vi "SUB-ROM Data convert to table.vi"(4 "ROM Table Ref":refnum<vi>, 5 "ROM Data Ref":refnum<vi>) -> (1 "ROM Table":string[][](table)=[["Device ID", "1 (00000001h)", "MAX Value: 4294967295 (FFFFFFFFh)"], ["YEAR", "2 (02h)", "Year: 2002, MAX Value: 255 (FFh)"], ["Month", "3 (03h)", "Month:  3, MAX Value: 255 (FFh)"], ["Day", "4 (04h)", "Day:  4, MAX Value: 255 (FFh)"], ["Device Type", "5 (0005h)", "-"], ["Manufacturer ID", "6 (00000006h)", "MAX Value: 4294967295 (FFFFFFFFh)"], ["Cal_Scale A", "7 (07h)", "MAX Value: 255 (FF)"], ["Cal_Scale B", "8 (08h)", "MAX Value: 255 (FF)"], ["Cal_Acc. X", "9 (0009h)", "-"], ["Cal_Acc. Y", "10 (000Ah)", "-"], ["Cal_Acc. Z", "11 (000Bh)", "-"], ["Cal_Gy. X", "12 (000Ch)", "-"], ["Cal_Gy. Y", "13 (000Dh)", "-"], ["Cal_Gy. Z", "14 (000Eh)", "-"], ["Cal_Vol H", "15 (000Fh)", "-"], ["Cal_Vol L", "16 (0010h)", "-"], ["Cal_CDC Off 1", "17 (11h)", "-"], ["Cal_CDC Off 2", "18 (12h)", "-"], ["Cal_CDC Off 3", "19 (13h)", "-"], ["Cal_CDC Off 4", "20 (14h)", "-"], ["Cal_CDC Off 5", "21 (15h)", "-"], ["Cal_CDC Off 6", "22 (16h)", "-"], ["Cal_CDC Off 7", "23 (17h)", "-"], ["Cal_CDC Off 8", "24 (18h)", "-"], ["Firmware Revision", "25 (19h)", "-"], ["Operative Side", "26 (1Ah)", "-"], ["Cal_Compart. A_10", "27 (0000001Bh)", "-"], ["Cal_Compart. B_10", "28 (0000001Ch)", "-"], ["Reserved", "29 (1Dh)", "-"], ["Cal_Compart. A_11", "30 (0000001Eh)", "-"], ["Cal_Compart. B_11", "31 (0000001Fh)", "-"], ["Cal_Compart. A_12", "32 (00000020h)", "-"], ["Cal_Compart. B_12", "33 (00000021h)", "-"], ["Cal_Compart. A_13", "34 (00000022h)", "-"], ["Cal_Compart. B_13", "35 (00000023h)", "-"], ["Cal_Compart. A_14", "36 (00000024h)", "-"], ["Cal_Compart. B_14", "37 (00000025h)", "-"], ["Cal_Compart. A_16", "38 (00000026h)", "-"], ["Cal_Compart. B_16", "39 (00000027h)", "-"], ["Reserved", "40 (28h)", "-"], ["Acc. X_0 value", "41 (0029h)", "-"], ["Acc. Y_0 value", "42 (002Ah)", "-"], ["Acc. Z_0 value", "43 (002Bh)", "-"], ["Acc. X_45 value", "44 (002Ch)", "-"], ["Acc. Y_45 value", "45 (002Dh)", "-"], ["Acc. Z_45 value", "46 (002Eh)", "-"], ["Reserved", "47 (2Fh)", "-"], ["Acc. X_90 value", "48 (0030h)", "-"], ["Acc. Y_90 value", "49 (0031h)", "-"], ["Acc. Z_90 value", "50 (0032h)", "-"], ["Acc. X_180 value", "51 (0033h)", "-"], ["Acc. Y_180 value", "52 (0034h)", "-"], ["Acc. Z_180 value", "53 (0035h)", "-"], ["Second counter", "16 (0000h)", "-"], ["Reserved", "54 (36h)", "-"], ["", "", ""], ["", "", ""], ["", "", ""], ["", "", ""], ["", "", ""], ["", "", ""], ["", "", ""], ["", "", ""], ["", "", ""], ["", "", ""], ["", "", ""], ["", "", ""], ["", "", ""], ["", "", ""], ["", "", ""]], 2 "ROM Data":T1(array[cluster])=[{"RxOK"=TRUE, "ROM Data"=[0, 0, 0, 1, 2, 3, 4, 0, 5, 0, 0, 0, 6, 7, 8, 131, 2], "Index"=0}, {"RxOK"=TRUE, "ROM Data"=[0, 9, 0, 10, 0, 11, 0, 12, 0, 13, 0, 14, 0, 15, 0, 136, 5], "Index"=1}, {"RxOK"=TRUE, "ROM Data"=[0, 17, 0, 18, 0, 19, 0, 20, 0, 21, 0, 22, 0, 23, 0, 145, 8], "Index"=2}, {"RxOK"=TRUE, "ROM Data"=[25, 26, 0, 0, 0, 27, 0, 0, 0, 28, 29, 0, 0, 0, 0, 146, 11], "Index"=3}, {"RxOK"=TRUE, "ROM Data"=[25, 26, 0, 0, 0, 27, 0, 0, 0, 28, 29, 0, 0, 0, 0, 146, 14], "Index"=4}, {"RxOK"=TRUE, "ROM Data"=[25, 26, 0, 0, 0, 27, 0, 0, 0, 28, 29, 0, 0, 0, 0, 146, 17], "Index"=5}, {"RxOK"=TRUE, "ROM Data"=[25, 26, 0, 0, 0, 27, 0, 0, 0, 28, 29, 0, 0, 0, 0, 146, 20], "Index"=6}, {"RxOK"=TRUE, "ROM Data"=[25, 26, 0, 0, 0, 27, 0, 0, 0, 28, 29, 0, 0, 0, 0, 146, 23], "Index"=7}, {"RxOK"=TRUE, "ROM Data"=[25, 26, 0, 0, 0, 27, 0, 0, 0, 28, 29, 0, 0, 0, 0, 146, 26], "Index"=8}] {"Index" format="%02x"; "ROM Data" format="%02x"})   [LabVIEW 2015]
panel:
  out "Last Index":i32=8
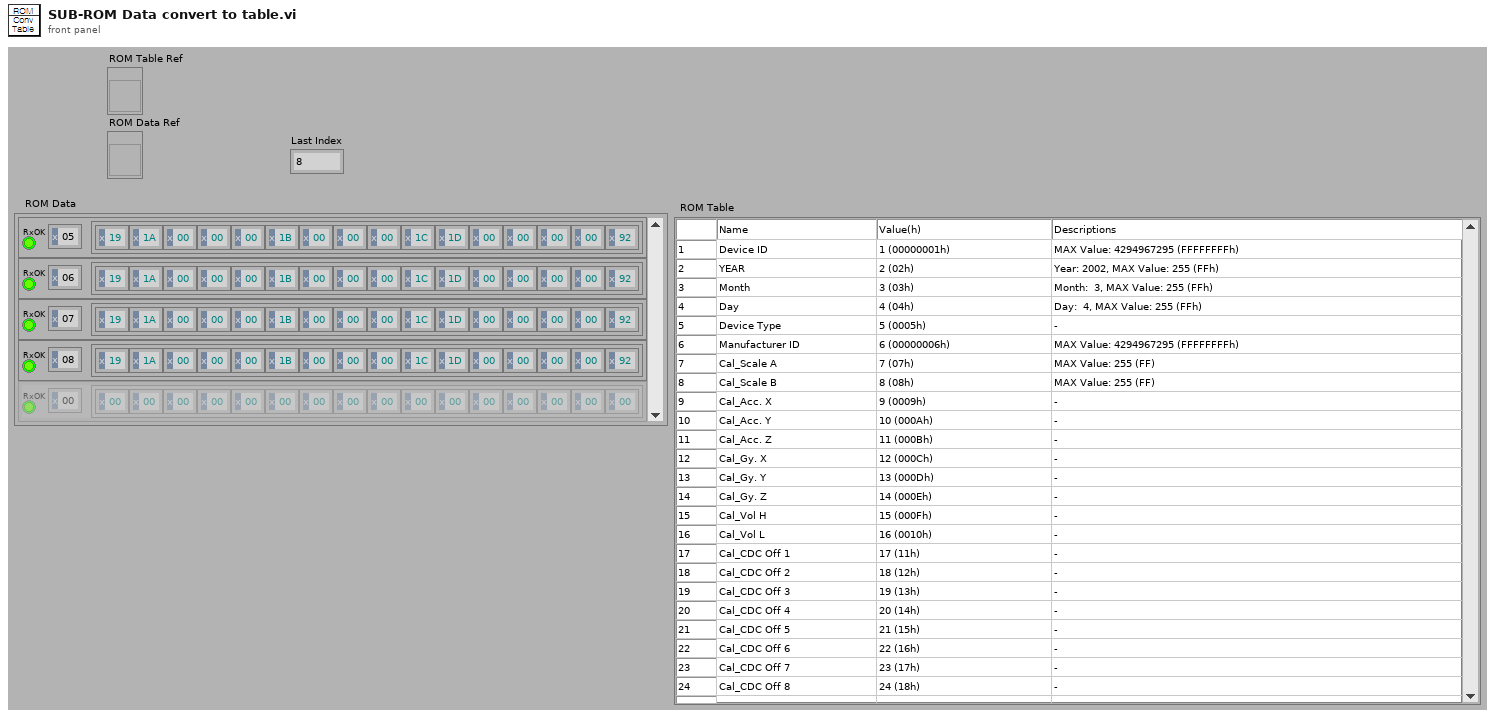
[diagram p1: front panel]
types:
  T1 = cluster{"RxOK":bool, "ROM Data":u8[], "Index":u8}[]
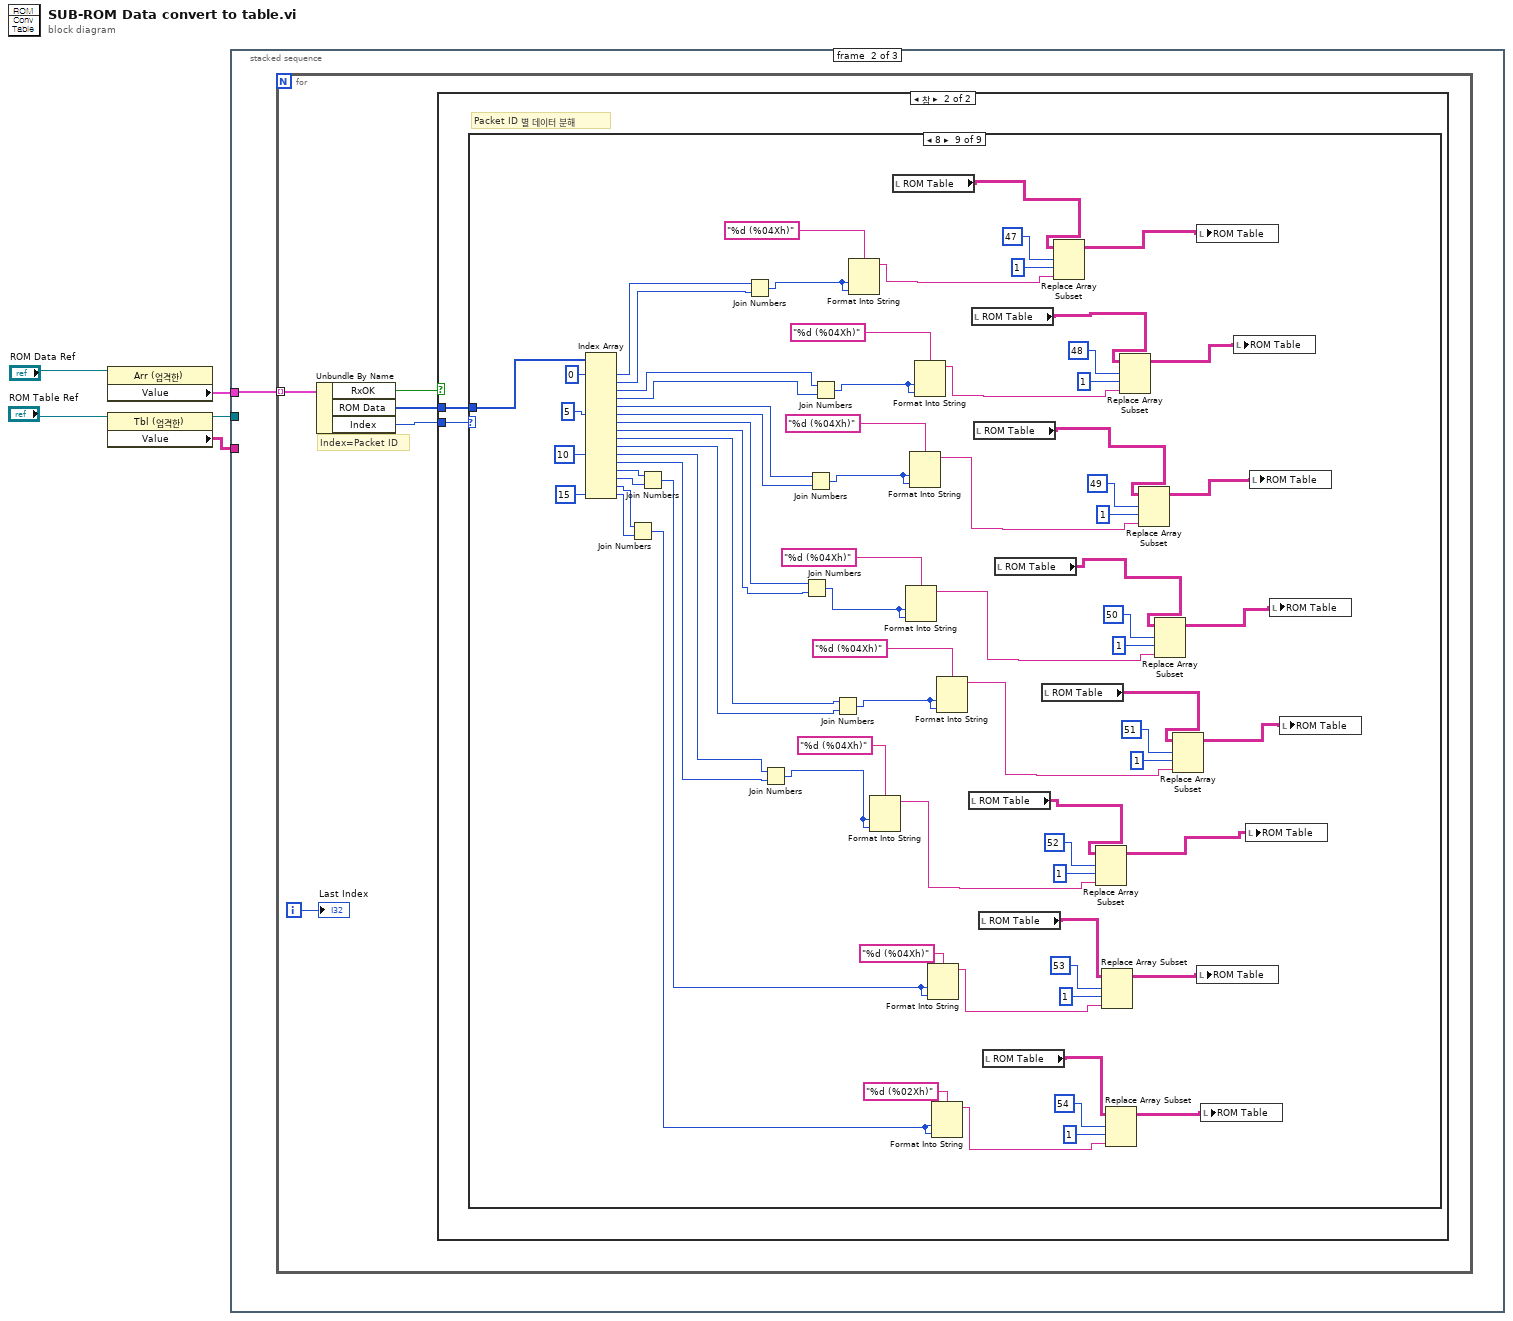
[diagram p0: block diagram]
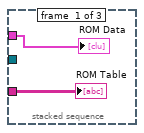
[diagram p2: hidden frame]
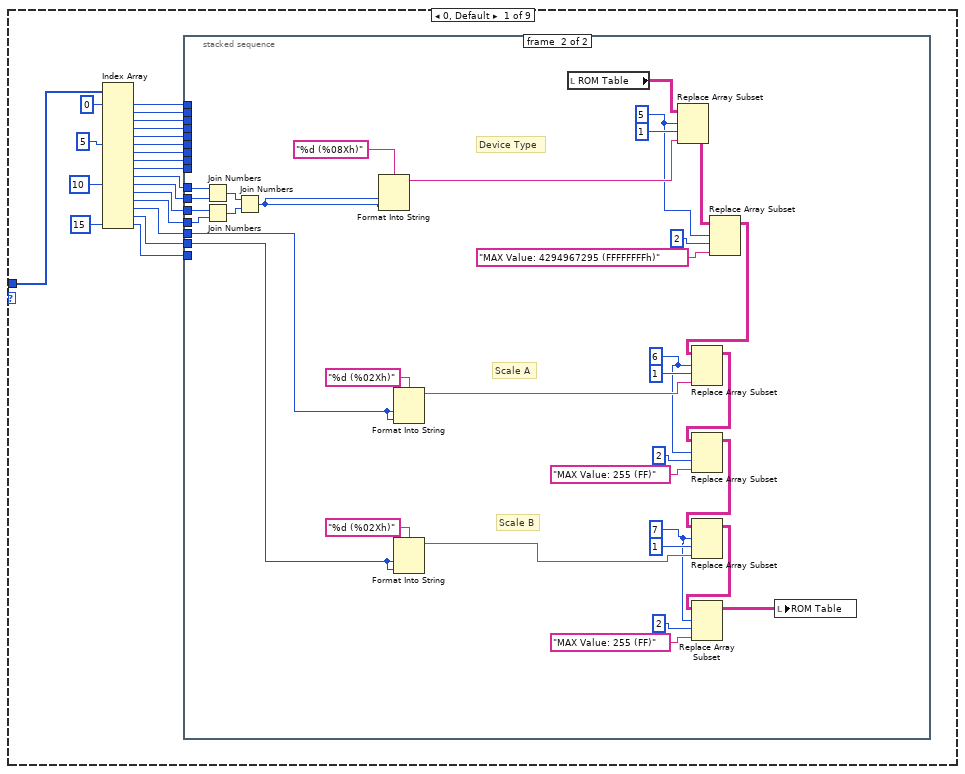
[diagram p4: hidden frame]
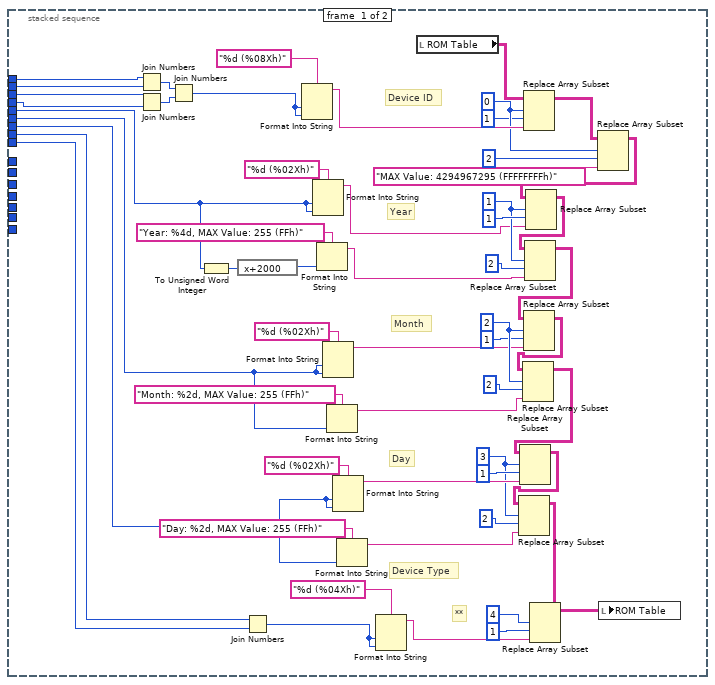
[diagram p5: hidden frame]
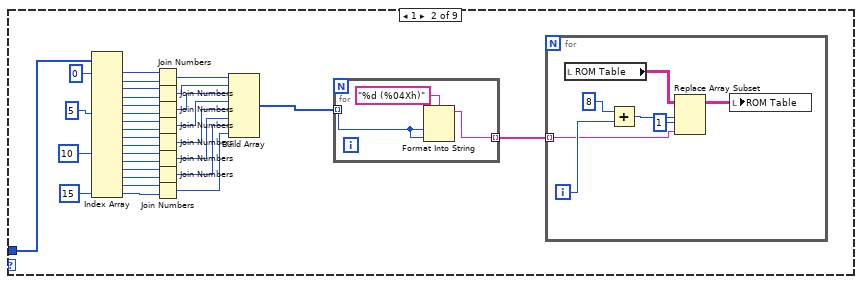
[diagram p6: hidden frame]
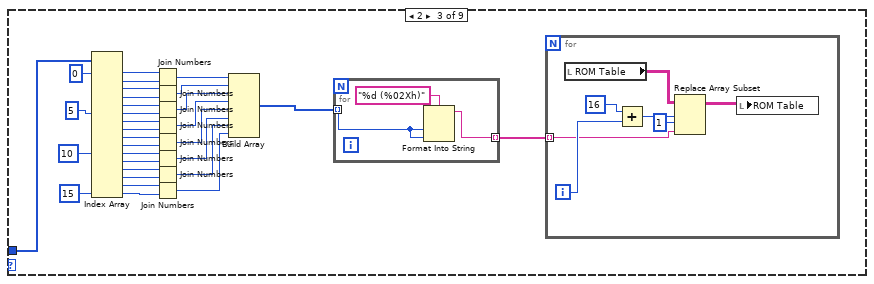
[diagram p7: hidden frame]
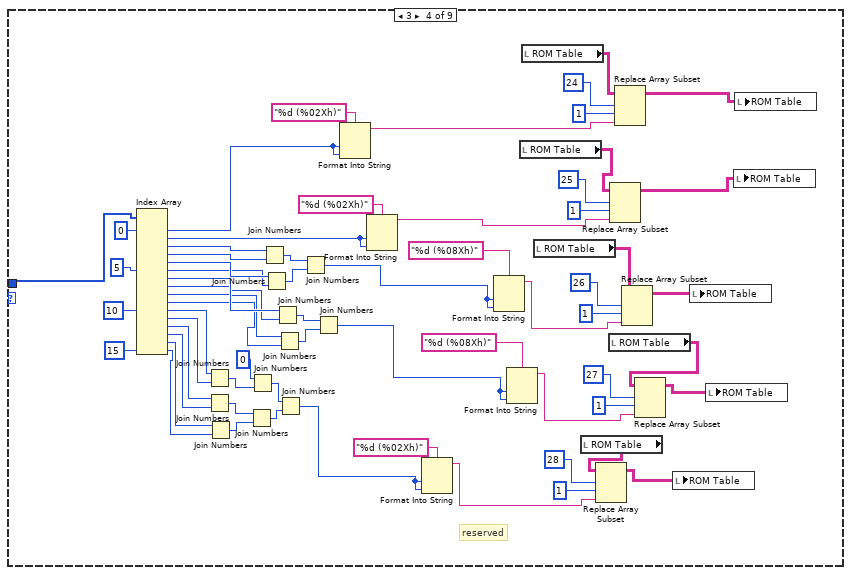
[diagram p8: hidden frame]
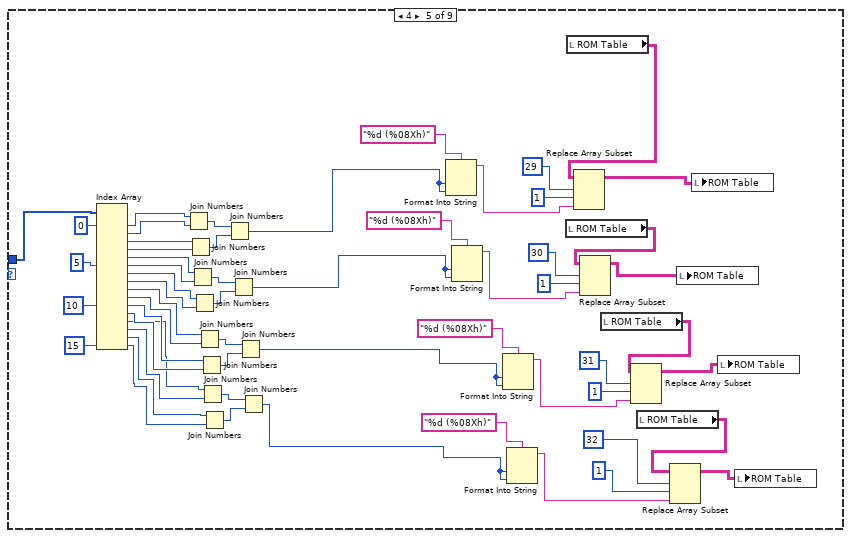
[diagram p9: hidden frame]
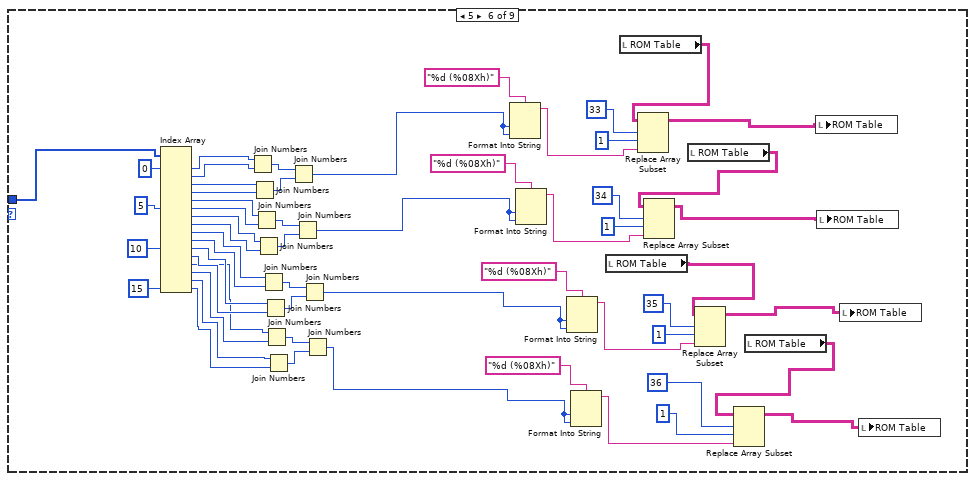
[diagram p10: hidden frame]
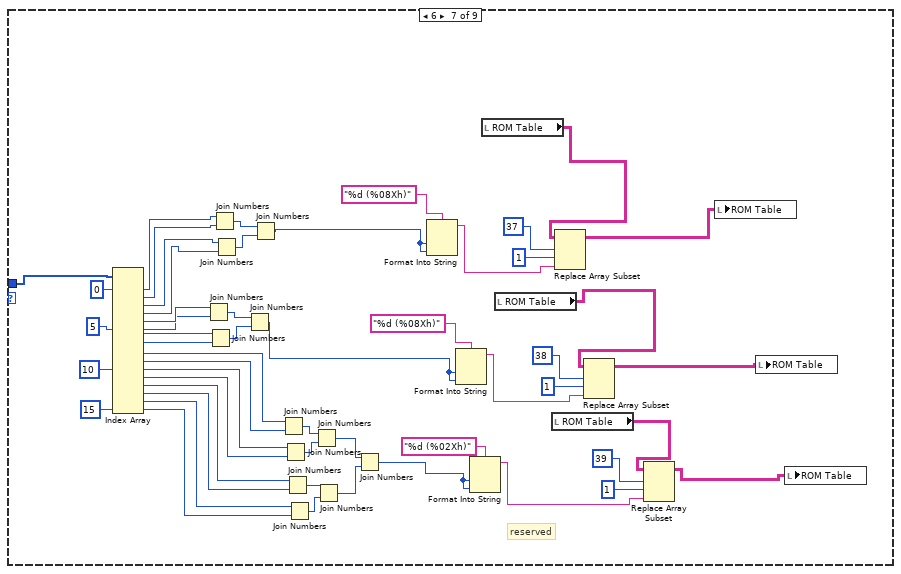
[diagram p11: hidden frame]
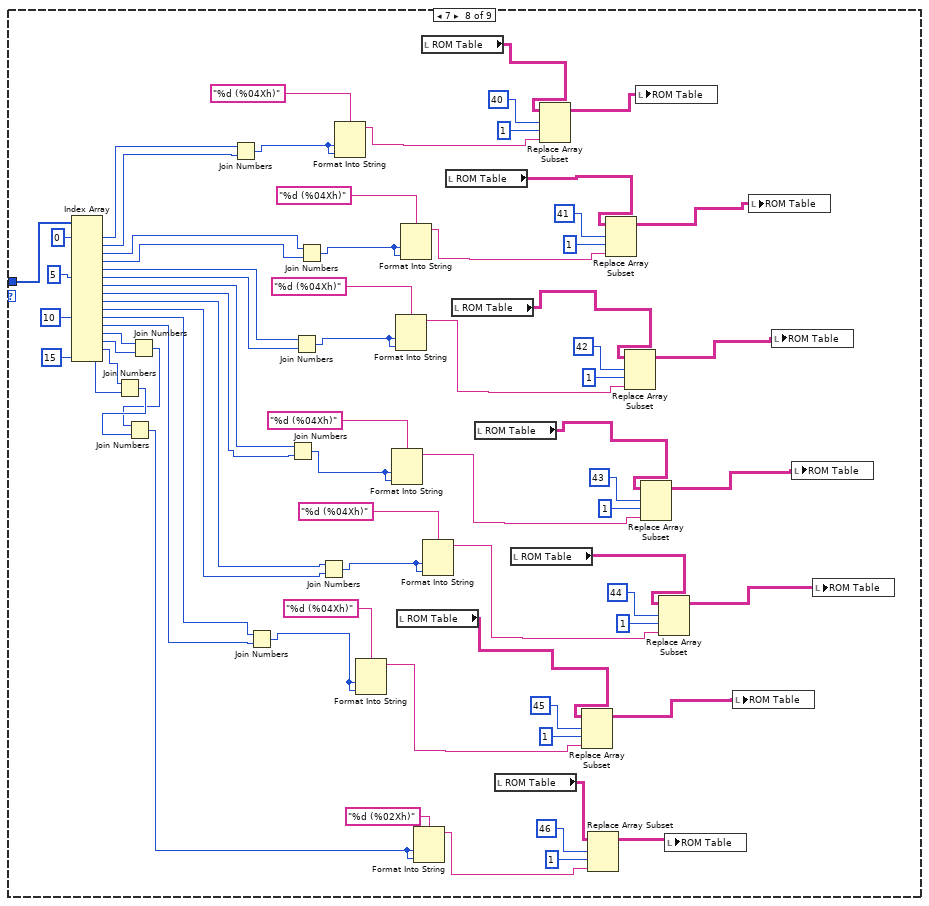
[diagram p12: hidden frame]
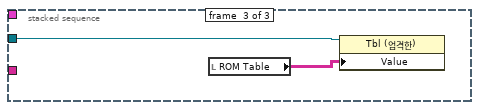
[diagram p13: hidden frame]
diagram:
  n1 = property class="Arr (엄격한)"(reference="ROM Data Ref") -> ("Value"=w3:T1)  [unwired: 1 in, 2 out]
  n2 = property class="Tbl (엄격한)"(reference="ROM Table Ref") -> (reference out=w1:refnum<vi>, "Value"=w2:string[][])  [unwired: 1 in, 1 out]
  n3 = stacked-sequence {
    tunnel: w3 -> [w7 w8 _]
    tunnel: w2 -> [w6 _ _]
    tunnel: w1 -> [_ _ w589]
    frame #0 {
      "ROM Data" <- w7
      "ROM Table" <- w6
    }
    frame #1 {
      n4 = for {
        tunnel: w8 -> [w13] mode=indexing
        i -> [w9]
        # "Index=Packet ID"
        n5 = Unbundle By Name(w13) -> ("RxOK"=w11:bool, "ROM Data"=w10:u8[], "Index"=w12:u8)
        n6 = case shown="참" w11 {
          tunnel: w12 -> [_ w15]
          tunnel: w10 -> [_ w14]
          frame False {
          }
          frame True {
            # "Packet ID 별 데이터 분해"
            n7 = case shown="8" w15 {
              tunnel: w14 -> [w32 w153 w194 w268 w325 w338 w434 w506 w537]
              frame 0, Default {
                n8 = Index Array(array=w32, index #1=0 ("인덱스"), index #6=5 ("인덱스"), index #11=10 ("인덱스"), index #16=15 ("인덱스")) -> (element #1=w31:u8, element #2=w30:u8, element #3=w29:u8, element #4=w28:u8, element #5=w27:u8, element #6=w26:u8, element #7=w25:u8, element #8=w24:u8, element #9=w23:u8, element #10=w22:u8, element #11=w21:u8, element #12=w20:u8, element #13=w19:u8, element #14=w18:u8, element #15=w17:u8, element #16=w16:u8)  [unwired: 12 in]
                n9 = stacked-sequence {
                  tunnel: w31 -> [w87 _]
                  tunnel: w30 -> [w86 _]
                  tunnel: w29 -> [w85 _]
                  tunnel: w28 -> [w84 _]
                  tunnel: w27 -> [w78 _]
                  tunnel: w26 -> [w64 _]
                  tunnel: w25 -> [w52 _]
                  tunnel: w24 -> [w46 _]
                  tunnel: w23 -> [w45 _]
                  tunnel: w22 -> [_ w124]
                  tunnel: w21 -> [_ w123]
                  tunnel: w20 -> [_ w122]
                  tunnel: w19 -> [_ w121]
                  tunnel: w18 -> [_ w113]
                  tunnel: w17 -> [_ w110]
                  tunnel: w16 -> [_ _]
                  frame #0 {
                    w56 = 3 ("인덱스 (행)")
                    w69 = 2 ("인덱스 (행)")
                    w75 = 1 ("인덱스 (행)")
                    w42 = 0 ("인덱스 (행)")
                    # "Device Type"
                    # "**"
                    # "Day"
                    # "Month"
                    # "Year"
                    # "Device ID"
                    n10 = Join Numbers(hi=w87, lo=w86) -> ((hi.lo)=w88:u16)
                    n11 = Join Numbers(hi=w85, lo=w84) -> ((hi.lo)=w89:u16)
                    n12 = Join Numbers(hi=w88, lo=w89) -> ((hi.lo)=w91:u32)
                    n13 = To Unsigned Word Integer(number=w78) -> (unsigned 16bit integer=w79:u16)
                    n14 = expression code="x+2000"(w79) -> (w80:u16)
                    n15 = Join Numbers(hi=w46, lo=w45) -> ((hi.lo)=w50:u16)
                    n16 = Format Into String(format string="%d (%08Xh)" ("포맷 문자열"), w91, w91) -> (resulting string=w83:string)  [unwired: 2 in, 1 out]
                    n17 = Format Into String(format string="%d (%02Xh)" ("포맷 문자열"), w78, w78) -> (resulting string=w73:string)  [unwired: 2 in, 1 out]
                    n18 = Format Into String(format string="Year: %4d, MAX Value: 255 (FFh)" ("포맷 문자열"), w80) -> (resulting string=w72:string)  [unwired: 2 in, 1 out]
                    n19 = Format Into String(format string="%d (%02Xh)" ("포맷 문자열"), w64, w64) -> (resulting string=w67:string)  [unwired: 2 in, 1 out]
                    n20 = Format Into String(format string="Month: %2d, MAX Value: 255 (FFh)" ("포맷 문자열"), w64) -> (resulting string=w71:string)  [unwired: 2 in, 1 out]
                    n21 = Format Into String(format string="%d (%02Xh)" ("포맷 문자열"), w52, w52) -> (resulting string=w59:string)  [unwired: 2 in, 1 out]
                    n22 = Format Into String(format string="Day: %2d, MAX Value: 255 (FFh)" ("포맷 문자열"), w52) -> (resulting string=w54:string)  [unwired: 2 in, 1 out]
                    n23 = Format Into String(format string="%d (%04Xh)" ("포맷 문자열"), w50, w50) -> (resulting string=w48:string)  [unwired: 2 in, 1 out]
                    n24 = local read "ROM Table"() -> (w92:string[][])
                    n25 = Replace Array Subset(array=w92, new element=w83, index (row)=w42, index (col)=1 ("비활성화된 인덱스 (열)")) -> (w44:string[][])
                    n26 = Replace Array Subset(array=w44, new element="MAX Value: 4294967295 (FFFFFFFFh)" ("새 원소/부분배열"), index (row)=w42, index (col)=2 ("비활성화된 인덱스 (열)")) -> (w43:string[][])
                    n27 = Replace Array Subset(array=w43, new element=w73, index (row)=w75, index (col)=1 ("인덱스 (행)")) -> (w74:string[][])
                    n28 = Replace Array Subset(array=w74, new element=w72, index (row)=w75, index (col)=2 ("인덱스 (행)")) -> (w63:string[][])
                    n29 = Replace Array Subset(array=w63, new element=w67, index (row)=w69, index (col)=1 ("인덱스 (행)")) -> (w62:string[][])
                    n30 = Replace Array Subset(array=w62, new element=w71, index (row)=w69, index (col)=2 ("인덱스 (행)")) -> (w53:string[][])
                    n31 = Replace Array Subset(array=w53, new element=w59, index (row)=w56, index (col)=1 ("인덱스 (행)")) -> (w57:string[][])
                    n32 = Replace Array Subset(array=w57, new element=w54, index (row)=w56, index (col)=2 ("인덱스 (행)")) -> (w47:string[][])
                    n33 = Replace Array Subset(array=w47, new element=w48, index (row)=4 ("인덱스 (행)"), index (col)=1 ("인덱스 (행)")) -> (w38:string[][])
                    n34 = local write "ROM Table"(w38) -> ()
                  }
                  frame #1 {
                    w99 = 7 ("인덱스 (행)")
                    w98 = 6 ("인덱스 (행)")
                    w93 = 5 ("인덱스 (행)")
                    # "Scale B"
                    # "Scale A"
                    # "Device Type"
                    n35 = Join Numbers(hi=w124, lo=w123) -> ((hi.lo)=w125:u16)
                    n36 = Join Numbers(hi=w122, lo=w121) -> ((hi.lo)=w126:u16)
                    n37 = Join Numbers(hi=w125, lo=w126) -> ((hi.lo)=w119:u32)
                    n38 = Format Into String(format string="%d (%08Xh)" ("포맷 문자열"), w119, w119) -> (resulting string=w116:string)  [unwired: 2 in, 1 out]
                    n39 = Format Into String(format string="%d (%02Xh)" ("포맷 문자열"), w113, w113) -> (resulting string=w112:string)  [unwired: 2 in, 1 out]
                    n40 = Format Into String(format string="%d (%02Xh)" ("포맷 문자열"), w110, w110) -> (resulting string=w108:string)  [unwired: 2 in, 1 out]
                    n41 = local read "ROM Table"() -> (w117:string[][])
                    n42 = Replace Array Subset(array=w117, new element=w116, index (row)=w93, index (col)=1 ("비활성화된 인덱스 (열)")) -> (w95:string[][])
                    n43 = Replace Array Subset(array=w95, new element="MAX Value: 4294967295 (FFFFFFFFh)" ("새 원소/부분배열"), index (row)=w93, index (col)=2 ("인덱스 (행)")) -> (w94:string[][])
                    n44 = Replace Array Subset(array=w94, new element=w112, index (row)=w98, index (col)=1 ("비활성화된 인덱스 (열)")) -> (w105:string[][])
                    n45 = Replace Array Subset(array=w105, new element="MAX Value: 255 (FF)" ("새 원소/부분배열"), index (row)=w98, index (col)=2 ("인덱스 (행)")) -> (w102:string[][])
                    n46 = Replace Array Subset(array=w102, new element=w108, index (row)=w99, index (col)=1 ("비활성화된 인덱스 (열)")) -> (w101:string[][])
                    n47 = Replace Array Subset(array=w101, new element="MAX Value: 255 (FF)" ("새 원소/부분배열"), index (row)=w99, index (col)=2 ("인덱스 (행)")) -> (w100:string[][])
                    n48 = local write "ROM Table"(w100) -> ()
                  }
                }
              }
              frame 1 {
                n49 = Index Array(array=w153, index #1=0 ("인덱스"), index #6=5 ("인덱스"), index #11=10 ("인덱스"), index #16=15 ("인덱스")) -> (element #1=w152:u8, element #2=w151:u8, element #3=w150:u8, element #4=w149:u8, element #5=w148:u8, element #6=w147:u8, element #7=w146:u8, element #8=w145:u8, element #9=w144:u8, element #10=w143:u8, element #11=w142:u8, element #12=w141:u8, element #13=w140:u8, element #14=w139:u8, element #15=w138:u8, element #16=w137:u8)  [unwired: 12 in]
                n50 = Join Numbers(hi=w152, lo=w151) -> ((hi.lo)=w136:u16)
                n51 = Join Numbers(hi=w150, lo=w149) -> ((hi.lo)=w135:u16)
                n52 = Join Numbers(hi=w148, lo=w147) -> ((hi.lo)=w134:u16)
                n53 = Join Numbers(hi=w146, lo=w145) -> ((hi.lo)=w133:u16)
                n54 = Join Numbers(hi=w144, lo=w143) -> ((hi.lo)=w132:u16)
                n55 = Join Numbers(hi=w142, lo=w141) -> ((hi.lo)=w131:u16)
                n56 = Join Numbers(hi=w140, lo=w139) -> ((hi.lo)=w130:u16)
                n57 = Join Numbers(hi=w138, lo=w137) -> ((hi.lo)=w129:u16)
                n58 = Build Array(w136, w135, w134, w133, w132, w131, w130, w129) -> (w128:u16[])
                n59 = for {
                  tunnel: w128 -> [w166] mode=indexing
                  tunnel: [w165] -> w127 mode=indexing
                  n60 = Format Into String(format string="%d (%04Xh)" ("포맷 문자열"), w166, w166) -> (resulting string=w165:string)  [unwired: 2 in, 1 out]
                }
                n61 = for {
                  tunnel: w127 -> [w161] mode=indexing
                  i -> [w162]
                  n62 = local read "ROM Table"() -> (w164:string[][])
                  n63 = Add(x=8, y=w162) -> (x+y=w159:i32)
                  n64 = Replace Array Subset(array=w164, new element=w161, index (row)=w159, index (col)=1 ("비활성화된 인덱스 (열)")) -> (w158:string[][])
                  n65 = local write "ROM Table"(w158) -> ()
                }
              }
              frame 2 {
                n66 = Index Array(array=w194, index #1=0 ("인덱스"), index #6=5 ("인덱스"), index #11=10 ("인덱스"), index #16=15 ("인덱스")) -> (element #1=w193:u8, element #2=w192:u8, element #3=w191:u8, element #4=w190:u8, element #5=w189:u8, element #6=w188:u8, element #7=w187:u8, element #8=w186:u8, element #9=w185:u8, element #10=w184:u8, element #11=w183:u8, element #12=w182:u8, element #13=w181:u8, element #14=w180:u8, element #15=w179:u8, element #16=w178:u8)  [unwired: 12 in]
                n67 = Join Numbers(hi=w193, lo=w192) -> ((hi.lo)=w177:u16)
                n68 = Join Numbers(hi=w191, lo=w190) -> ((hi.lo)=w176:u16)
                n69 = Join Numbers(hi=w189, lo=w188) -> ((hi.lo)=w175:u16)
                n70 = Join Numbers(hi=w187, lo=w186) -> ((hi.lo)=w174:u16)
                n71 = Join Numbers(hi=w185, lo=w184) -> ((hi.lo)=w173:u16)
                n72 = Join Numbers(hi=w183, lo=w182) -> ((hi.lo)=w172:u16)
                n73 = Join Numbers(hi=w181, lo=w180) -> ((hi.lo)=w171:u16)
                n74 = Join Numbers(hi=w179, lo=w178) -> ((hi.lo)=w170:u16)
                n75 = Build Array(w177, w176, w175, w174, w173, w172, w171, w170) -> (w169:u16[])
                n76 = for {
                  tunnel: w169 -> [w207] mode=indexing
                  tunnel: [w206] -> w168 mode=indexing
                  n77 = Format Into String(format string="%d (%02Xh)" ("포맷 문자열"), w207, w207) -> (resulting string=w206:string)  [unwired: 2 in, 1 out]
                }
                n78 = for {
                  tunnel: w168 -> [w202] mode=indexing
                  i -> [w203]
                  n79 = local read "ROM Table"() -> (w205:string[][])
                  n80 = Add(x=16, y=w203) -> (x+y=w200:i32)
                  n81 = Replace Array Subset(array=w205, new element=w202, index (row)=w200, index (col)=1 ("비활성화된 인덱스 (열)")) -> (w199:string[][])
                  n82 = local write "ROM Table"(w199) -> ()
                }
              }
              frame 3 {
                # "reserved"
                n83 = Index Array(array=w268, index #1=0 ("인덱스"), index #6=5 ("인덱스"), index #11=10 ("인덱스"), index #16=15 ("인덱스")) -> (element #1=w266:u8, element #2=w259:u8, element #3=w253:u8, element #4=w252:u8, element #5=w251:u8, element #6=w250:u8, element #7=w233:u8, element #8=w232:u8, element #9=w231:u8, element #10=w230:u8, element #11=w214:u8, element #12=w213:u8, element #13=w212:u8, element #14=w211:u8, element #15=w210:u8, element #16=w209:u8)  [unwired: 12 in]
                n84 = Join Numbers(hi=w214, lo=w213) -> ((hi.lo)=w217:u16)
                n85 = Join Numbers(hi=w212, lo=w211) -> ((hi.lo)=w220:u16)
                n86 = Join Numbers(hi=w210, lo=w209) -> ((hi.lo)=w221:u16)
                n87 = Join Numbers(hi=w220, lo=w221) -> ((hi.lo)=w218:u32)
                n88 = Join Numbers(hi=u16 0, lo=w217) -> ((hi.lo)=w219:u32)
                n89 = Join Numbers(hi=w253, lo=w252) -> ((hi.lo)=w249:u16)
                n90 = Join Numbers(hi=w251, lo=w250) -> ((hi.lo)=w248:u16)
                n91 = Join Numbers(hi=w233, lo=w232) -> ((hi.lo)=w240:u16)
                n92 = Join Numbers(hi=w231, lo=w230) -> ((hi.lo)=w239:u16)
                n93 = Join Numbers(hi=w219, lo=w218) -> ((hi.lo)=w215:u64)
                n94 = Join Numbers(hi=w249, lo=w248) -> ((hi.lo)=w246:u32)
                n95 = Join Numbers(hi=w240, lo=w239) -> ((hi.lo)=w237:u32)
                n96 = Format Into String(format string="%d (%02Xh)" ("포맷 문자열"), w266, w266) -> (resulting string=w262:string)  [unwired: 2 in, 1 out]
                n97 = Format Into String(format string="%d (%02Xh)" ("포맷 문자열"), w259, w259) -> (resulting string=w254:string)  [unwired: 2 in, 1 out]
                n98 = Format Into String(format string="%d (%02Xh)" ("포맷 문자열"), w215, w215) -> (resulting string=w224:string)  [unwired: 2 in, 1 out]
                n99 = Format Into String(format string="%d (%08Xh)" ("포맷 문자열"), w246, w246) -> (resulting string=w241:string)  [unwired: 2 in, 1 out]
                n100 = Format Into String(format string="%d (%08Xh)" ("포맷 문자열"), w237, w237) -> (resulting string=w234:string)  [unwired: 2 in, 1 out]
                n101 = local read "ROM Table"() -> (w256:string[][])
                n102 = local read "ROM Table"() -> (w264:string[][])
                n103 = local read "ROM Table"() -> (w243:string[][])
                n104 = local read "ROM Table"() -> (w223:string[][])
                n105 = Replace Array Subset(array=w223, new element=w224, index (row)=28 ("비활성화된 인덱스 (열)"), index (col)=1 ("비활성화된 인덱스 (열)")) -> (w222:string[][])
                n106 = local read "ROM Table"() -> (w229:string[][])
                n107 = Replace Array Subset(array=w256, new element=w254, index (row)=25 ("비활성화된 인덱스 (열)"), index (col)=1 ("비활성화된 인덱스 (열)")) -> (w255:string[][])
                n108 = Replace Array Subset(array=w264, new element=w262, index (row)=24 ("비활성화된 인덱스 (열)"), index (col)=1 ("비활성화된 인덱스 (열)")) -> (w261:string[][])
                n109 = Replace Array Subset(array=w243, new element=w241, index (row)=26 ("비활성화된 인덱스 (열)"), index (col)=1 ("비활성화된 인덱스 (열)")) -> (w242:string[][])
                n110 = Replace Array Subset(array=w229, new element=w234, index (row)=27 ("비활성화된 인덱스 (열)"), index (col)=1 ("비활성화된 인덱스 (열)")) -> (w228:string[][])
                n111 = local write "ROM Table"(w222) -> ()
                n112 = local write "ROM Table"(w242) -> ()
                n113 = local write "ROM Table"(w228) -> ()
                n114 = local write "ROM Table"(w255) -> ()
                n115 = local write "ROM Table"(w261) -> ()
              }
              frame 4 {
                n116 = Index Array(array=w325, index #1=0 ("인덱스"), index #6=5 ("인덱스"), index #11=10 ("인덱스"), index #16=15 ("인덱스")) -> (element #1=w295:u8, element #2=w294:u8, element #3=w293:u8, element #4=w292:u8, element #5=w291:u8, element #6=w290:u8, element #7=w289:u8, element #8=w288:u8, element #9=w287:u8, element #10=w286:u8, element #11=w285:u8, element #12=w284:u8, element #13=w283:u8, element #14=w273:u8, element #15=w282:u8, element #16=w281:u8)  [unwired: 12 in]
                n117 = Join Numbers(hi=w295, lo=w294) -> ((hi.lo)=w324:u16)
                n118 = Join Numbers(hi=w293, lo=w292) -> ((hi.lo)=w323:u16)
                n119 = Join Numbers(hi=w291, lo=w290) -> ((hi.lo)=w315:u16)
                n120 = Join Numbers(hi=w289, lo=w288) -> ((hi.lo)=w314:u16)
                n121 = Join Numbers(hi=w287, lo=w286) -> ((hi.lo)=w306:u16)
                n122 = Join Numbers(hi=w285, lo=w284) -> ((hi.lo)=w305:u16)
                n123 = Join Numbers(hi=w283, lo=w273) -> ((hi.lo)=w297:u16)
                n124 = Join Numbers(hi=w282, lo=w281) -> ((hi.lo)=w296:u16)
                n125 = Join Numbers(hi=w324, lo=w323) -> ((hi.lo)=w322:u32)
                n126 = Join Numbers(hi=w315, lo=w314) -> ((hi.lo)=w313:u32)
                n127 = Join Numbers(hi=w306, lo=w305) -> ((hi.lo)=w301:u32)
                n128 = Join Numbers(hi=w297, lo=w296) -> ((hi.lo)=w278:u32)
                n129 = Format Into String(format string="%d (%08Xh)" ("포맷 문자열"), w322, w322) -> (resulting string=w319:string)  [unwired: 2 in, 1 out]
                n130 = Format Into String(format string="%d (%08Xh)" ("포맷 문자열"), w313, w313) -> (resulting string=w310:string)  [unwired: 2 in, 1 out]
                n131 = Format Into String(format string="%d (%08Xh)" ("포맷 문자열"), w301, w301) -> (resulting string=w300:string)  [unwired: 2 in, 1 out]
                n132 = Format Into String(format string="%d (%08Xh)" ("포맷 문자열"), w278, w278) -> (resulting string=w279:string)  [unwired: 2 in, 1 out]
                n133 = local read "ROM Table"() -> (w307:string[][])
                n134 = local read "ROM Table"() -> (w317:string[][])
                n135 = Replace Array Subset(array=w317, new element=w319, index (row)=29 ("비활성화된 인덱스 (열)"), index (col)=1 ("비활성화된 인덱스 (열)")) -> (w316:string[][])
                n136 = Replace Array Subset(array=w307, new element=w310, index (row)=30 ("비활성화된 인덱스 (열)"), index (col)=1 ("비활성화된 인덱스 (열)")) -> (w308:string[][])
                n137 = local read "ROM Table"() -> (w299:string[][])
                n138 = Replace Array Subset(array=w299, new element=w300, index (row)=31 ("비활성화된 인덱스 (열)"), index (col)=1 ("비활성화된 인덱스 (열)")) -> (w298:string[][])
                n139 = local read "ROM Table"() -> (w277:string[][])
                n140 = Replace Array Subset(array=w277, new element=w279, index (row)=32 ("비활성화된 인덱스 (열)"), index (col)=1 ("비활성화된 인덱스 (열)")) -> (w276:string[][])
                n141 = local write "ROM Table"(w308) -> ()
                n142 = local write "ROM Table"(w316) -> ()
                n143 = local write "ROM Table"(w298) -> ()
                n144 = local write "ROM Table"(w276) -> ()
              }
              frame 5 {
                n145 = Index Array(array=w338, index #1=0 ("인덱스"), index #6=5 ("인덱스"), index #11=10 ("인덱스"), index #16=15 ("인덱스")) -> (element #1=w359:u8, element #2=w358:u8, element #3=w357:u8, element #4=w356:u8, element #5=w355:u8, element #6=w354:u8, element #7=w353:u8, element #8=w352:u8, element #9=w351:u8, element #10=w350:u8, element #11=w349:u8, element #12=w348:u8, element #13=w347:u8, element #14=w346:u8, element #15=w345:u8, element #16=w344:u8)  [unwired: 12 in]
                n146 = Join Numbers(hi=w359, lo=w358) -> ((hi.lo)=w382:u16)
                n147 = Join Numbers(hi=w357, lo=w356) -> ((hi.lo)=w381:u16)
                n148 = Join Numbers(hi=w355, lo=w354) -> ((hi.lo)=w375:u16)
                n149 = Join Numbers(hi=w353, lo=w352) -> ((hi.lo)=w374:u16)
                n150 = Join Numbers(hi=w351, lo=w350) -> ((hi.lo)=w368:u16)
                n151 = Join Numbers(hi=w349, lo=w348) -> ((hi.lo)=w367:u16)
                n152 = Join Numbers(hi=w347, lo=w346) -> ((hi.lo)=w361:u16)
                n153 = Join Numbers(hi=w345, lo=w344) -> ((hi.lo)=w360:u16)
                n154 = Join Numbers(hi=w382, lo=w381) -> ((hi.lo)=w380:u32)
                n155 = Join Numbers(hi=w375, lo=w374) -> ((hi.lo)=w373:u32)
                n156 = Join Numbers(hi=w368, lo=w367) -> ((hi.lo)=w363:u32)
                n157 = Join Numbers(hi=w361, lo=w360) -> ((hi.lo)=w341:u32)
                n158 = Format Into String(format string="%d (%08Xh)" ("포맷 문자열"), w380, w380) -> (resulting string=w377:string)  [unwired: 2 in, 1 out]
                n159 = Format Into String(format string="%d (%08Xh)" ("포맷 문자열"), w373, w373) -> (resulting string=w370:string)  [unwired: 2 in, 1 out]
                n160 = Format Into String(format string="%d (%08Xh)" ("포맷 문자열"), w363, w363) -> (resulting string=w362:string)  [unwired: 2 in, 1 out]
                n161 = Format Into String(format string="%d (%08Xh)" ("포맷 문자열"), w341, w341) -> (resulting string=w342:string)  [unwired: 2 in, 1 out]
                n162 = local read "ROM Table"() -> (w331:string[][])
                n163 = local read "ROM Table"() -> (w333:string[][])
                n164 = Replace Array Subset(array=w333, new element=w377, index (row)=33 ("비활성화된 인덱스 (열)"), index (col)=1 ("비활성화된 인덱스 (열)")) -> (w334:string[][])
                n165 = local read "ROM Table"() -> (w332:string[][])
                n166 = Replace Array Subset(array=w332, new element=w370, index (row)=34 ("비활성화된 인덱스 (열)"), index (col)=1 ("비활성화된 인덱스 (열)")) -> (w335:string[][])
                n167 = Replace Array Subset(array=w331, new element=w362, index (row)=35 ("비활성화된 인덱스 (열)"), index (col)=1 ("비활성화된 인덱스 (열)")) -> (w336:string[][])
                n168 = local read "ROM Table"() -> (w330:string[][])
                n169 = Replace Array Subset(array=w330, new element=w342, index (row)=36 ("비활성화된 인덱스 (열)"), index (col)=1 ("비활성화된 인덱스 (열)")) -> (w337:string[][])
                n170 = local write "ROM Table"(w334) -> ()
                n171 = local write "ROM Table"(w335) -> ()
                n172 = local write "ROM Table"(w336) -> ()
                n173 = local write "ROM Table"(w337) -> ()
              }
              frame 6 {
                # "reserved"
                n174 = Index Array(array=w434, index #1=0 ("인덱스"), index #6=5 ("인덱스"), index #11=10 ("인덱스"), index #16=15 ("인덱스")) -> (element #1=w415:u8, element #2=w414:u8, element #3=w413:u8, element #4=w412:u8, element #5=w411:u8, element #6=w410:u8, element #7=w409:u8, element #8=w408:u8, element #9=w394:u8, element #10=w393:u8, element #11=w392:u8, element #12=w391:u8, element #13=w390:u8, element #14=w389:u8, element #15=w388:u8, element #16=w387:u8)  [unwired: 12 in]
                n175 = Join Numbers(hi=w411, lo=w410) -> ((hi.lo)=w424:u16)
                n176 = Join Numbers(hi=w409, lo=w408) -> ((hi.lo)=w423:u16)
                n177 = Join Numbers(hi=w415, lo=w414) -> ((hi.lo)=w433:u16)
                n178 = Join Numbers(hi=w413, lo=w412) -> ((hi.lo)=w432:u16)
                n179 = Join Numbers(hi=w424, lo=w423) -> ((hi.lo)=w418:u32)
                n180 = Join Numbers(hi=w433, lo=w432) -> ((hi.lo)=w427:u32)
                n181 = Join Numbers(hi=w394, lo=w393) -> ((hi.lo)=w401:u16)
                n182 = Join Numbers(hi=w392, lo=w391) -> ((hi.lo)=w400:u16)
                n183 = Join Numbers(hi=w390, lo=w389) -> ((hi.lo)=w399:u16)
                n184 = Join Numbers(hi=w388, lo=w387) -> ((hi.lo)=w398:u16)
                n185 = Join Numbers(hi=w401, lo=w400) -> ((hi.lo)=w397:u32)
                n186 = Join Numbers(hi=w399, lo=w398) -> ((hi.lo)=w396:u32)
                n187 = Join Numbers(hi=w397, lo=w396) -> ((hi.lo)=w395:u64)
                n188 = Format Into String(format string="%d (%08Xh)" ("포맷 문자열"), w427, w427) -> (resulting string=w429:string)  [unwired: 2 in, 1 out]
                n189 = Format Into String(format string="%d (%08Xh)" ("포맷 문자열"), w418, w418) -> (resulting string=w420:string)  [unwired: 2 in, 1 out]
                n190 = Format Into String(format string="%d (%02Xh)" ("포맷 문자열"), w395, w395) -> (resulting string=w404:string)  [unwired: 2 in, 1 out]
                n191 = local read "ROM Table"() -> (w426:string[][])
                n192 = local read "ROM Table"() -> (w417:string[][])
                n193 = local read "ROM Table"() -> (w403:string[][])
                n194 = Replace Array Subset(array=w426, new element=w429, index (row)=37 ("비활성화된 인덱스 (열)"), index (col)=1 ("비활성화된 인덱스 (열)")) -> (w425:string[][])
                n195 = Replace Array Subset(array=w417, new element=w420, index (row)=38 ("비활성화된 인덱스 (열)"), index (col)=1 ("비활성화된 인덱스 (열)")) -> (w416:string[][])
                n196 = Replace Array Subset(array=w403, new element=w404, index (row)=39 ("비활성화된 인덱스 (열)"), index (col)=1 ("비활성화된 인덱스 (열)")) -> (w402:string[][])
                n197 = local write "ROM Table"(w425) -> ()
                n198 = local write "ROM Table"(w416) -> ()
                n199 = local write "ROM Table"(w402) -> ()
              }
              frame 7 {
                n200 = Index Array(array=w506, index #1=0 ("인덱스"), index #6=5 ("인덱스"), index #11=10 ("인덱스"), index #16=15 ("인덱스")) -> (element #1=w463:u8, element #2=w462:u8, element #3=w461:u8, element #4=w460:u8, element #5=w459:u8, element #6=w458:u8, element #7=w457:u8, element #8=w456:u8, element #9=w455:u8, element #10=w454:u8, element #11=w453:u8, element #12=w452:u8, element #13=w445:u8, element #14=w444:u8, element #15=w443:u8, element #16=w442:u8)  [unwired: 12 in]
                n201 = Join Numbers(hi=w443, lo=w442) -> ((hi.lo)=w441:u16)
                n202 = Join Numbers(hi=w445, lo=w444) -> ((hi.lo)=w440:u16)
                n203 = Join Numbers(hi=w440, lo=w441) -> ((hi.lo)=w439:u32)
                n204 = Join Numbers(hi=w463, lo=w462) -> ((hi.lo)=w499:u16)
                n205 = Join Numbers(hi=w453, lo=w452) -> ((hi.lo)=w474:u16)
                n206 = Join Numbers(hi=w457, lo=w456) -> ((hi.lo)=w484:u16)
                n207 = Join Numbers(hi=w459, lo=w458) -> ((hi.lo)=w489:u16)
                n208 = Join Numbers(hi=w461, lo=w460) -> ((hi.lo)=w494:u16)
                n209 = Join Numbers(hi=w455, lo=w454) -> ((hi.lo)=w479:u16)
                n210 = Format Into String(format string="%d (%04Xh)" ("포맷 문자열"), w499, w499) -> (resulting string=w500:string)  [unwired: 2 in, 1 out]
                n211 = Format Into String(format string="%d (%04Xh)" ("포맷 문자열"), w474, w474) -> (resulting string=w475:string)  [unwired: 2 in, 1 out]
                n212 = Format Into String(format string="%d (%04Xh)" ("포맷 문자열"), w484, w484) -> (resulting string=w485:string)  [unwired: 2 in, 1 out]
                n213 = Format Into String(format string="%d (%04Xh)" ("포맷 문자열"), w489, w489) -> (resulting string=w490:string)  [unwired: 2 in, 1 out]
                n214 = local read "ROM Table"() -> (w466:string[][])
                n215 = Format Into String(format string="%d (%04Xh)" ("포맷 문자열"), w494, w494) -> (resulting string=w495:string)  [unwired: 2 in, 1 out]
                n216 = Format Into String(format string="%d (%02Xh)" ("포맷 문자열"), w439, w439) -> (resulting string=w448:string)  [unwired: 2 in, 1 out]
                n217 = local read "ROM Table"() -> (w503:string[][])
                n218 = Format Into String(format string="%d (%04Xh)" ("포맷 문자열"), w479, w479) -> (resulting string=w480:string)  [unwired: 2 in, 1 out]
                n219 = local read "ROM Table"() -> (w473:string[][])
                n220 = local read "ROM Table"() -> (w471:string[][])
                n221 = local read "ROM Table"() -> (w469:string[][])
                n222 = local read "ROM Table"() -> (w447:string[][])
                n223 = local read "ROM Table"() -> (w464:string[][])
                n224 = Replace Array Subset(array=w503, new element=w500, index (row)=40 ("비활성화된 인덱스 (열)"), index (col)=1 ("비활성화된 인덱스 (열)")) -> (w502:string[][])
                n225 = Replace Array Subset(array=w466, new element=w475, index (row)=45 ("비활성화된 인덱스 (열)"), index (col)=1 ("비활성화된 인덱스 (열)")) -> (w465:string[][])
                n226 = Replace Array Subset(array=w447, new element=w448, index (row)=46 ("비활성화된 인덱스 (열)"), index (col)=1 ("비활성화된 인덱스 (열)")) -> (w446:string[][])
                n227 = Replace Array Subset(array=w473, new element=w495, index (row)=41 ("비활성화된 인덱스 (열)"), index (col)=1 ("비활성화된 인덱스 (열)")) -> (w472:string[][])
                n228 = Replace Array Subset(array=w471, new element=w490, index (row)=42 ("비활성화된 인덱스 (열)"), index (col)=1 ("비활성화된 인덱스 (열)")) -> (w470:string[][])
                n229 = local write "ROM Table"(w502) -> ()
                n230 = Replace Array Subset(array=w469, new element=w485, index (row)=43 ("비활성화된 인덱스 (열)"), index (col)=1 ("비활성화된 인덱스 (열)")) -> (w468:string[][])
                n231 = Replace Array Subset(array=w464, new element=w480, index (row)=44 ("비활성화된 인덱스 (열)"), index (col)=1 ("비활성화된 인덱스 (열)")) -> (w467:string[][])
                n232 = local write "ROM Table"(w446) -> ()
                n233 = local write "ROM Table"(w465) -> ()
                n234 = local write "ROM Table"(w472) -> ()
                n235 = local write "ROM Table"(w470) -> ()
                n236 = local write "ROM Table"(w468) -> ()
                n237 = local write "ROM Table"(w467) -> ()
              }
              frame 8 {
                n238 = Index Array(array=w537, index #1=0 ("인덱스"), index #6=5 ("인덱스"), index #11=10 ("인덱스"), index #16=15 ("인덱스")) -> (element #1=w553:u8, element #2=w552:u8, element #3=w551:u8, element #4=w550:u8, element #5=w549:u8, element #6=w548:u8, element #7=w547:u8, element #8=w546:u8, element #9=w545:u8, element #10=w544:u8, element #11=w543:u8, element #12=w542:u8, element #13=w516:u8, element #14=w515:u8, element #15=w514:u8, element #16=w513:u8)  [unwired: 12 in]
                n239 = Join Numbers(hi=w514, lo=w513) -> ((hi.lo)=w512:u16)
                n240 = Join Numbers(hi=w516, lo=w515) -> ((hi.lo)=w511:u16)
                n241 = Join Numbers(hi=w553, lo=w552) -> ((hi.lo)=w579:u16)
                n242 = Join Numbers(hi=w543, lo=w542) -> ((hi.lo)=w554:u16)
                n243 = Join Numbers(hi=w547, lo=w546) -> ((hi.lo)=w564:u16)
                n244 = Join Numbers(hi=w549, lo=w548) -> ((hi.lo)=w569:u16)
                n245 = Join Numbers(hi=w551, lo=w550) -> ((hi.lo)=w574:u16)
                n246 = Join Numbers(hi=w545, lo=w544) -> ((hi.lo)=w559:u16)
                n247 = Format Into String(format string="%d (%04Xh)" ("포맷 문자열"), w579, w579) -> (resulting string=w580:string)  [unwired: 2 in, 1 out]
                n248 = Format Into String(format string="%d (%04Xh)" ("포맷 문자열"), w554, w554) -> (resulting string=w555:string)  [unwired: 2 in, 1 out]
                n249 = local read "ROM Table"() -> (w536:string[][])
                n250 = Format Into String(format string="%d (%04Xh)" ("포맷 문자열"), w564, w564) -> (resulting string=w565:string)  [unwired: 2 in, 1 out]
                n251 = Format Into String(format string="%d (%04Xh)" ("포맷 문자열"), w569, w569) -> (resulting string=w570:string)  [unwired: 2 in, 1 out]
                n252 = Format Into String(format string="%d (%04Xh)" ("포맷 문자열"), w574, w574) -> (resulting string=w575:string)  [unwired: 2 in, 1 out]
                n253 = Format Into String(format string="%d (%04Xh)" ("포맷 문자열"), w511, w511) -> (resulting string=w538:string)  [unwired: 2 in, 1 out]
                n254 = Format Into String(format string="%d (%02Xh)" ("포맷 문자열"), w512, w512) -> (resulting string=w520:string)  [unwired: 2 in, 1 out]
                n255 = Format Into String(format string="%d (%04Xh)" ("포맷 문자열"), w559, w559) -> (resulting string=w560:string)  [unwired: 2 in, 1 out]
                n256 = local read "ROM Table"() -> (w526:string[][])
                n257 = local read "ROM Table"() -> (w534:string[][])
                n258 = local read "ROM Table"() -> (w532:string[][])
                n259 = local read "ROM Table"() -> (w524:string[][])
                n260 = local read "ROM Table"() -> (w521:string[][])
                n261 = local read "ROM Table"() -> (w530:string[][])
                n262 = local read "ROM Table"() -> (w528:string[][])
                n263 = Replace Array Subset(array=w536, new element=w580, index (row)=47 ("비활성화된 인덱스 (열)"), index (col)=1 ("비활성화된 인덱스 (열)")) -> (w535:string[][])
                n264 = Replace Array Subset(array=w526, new element=w555, index (row)=52 ("비활성화된 인덱스 (열)"), index (col)=1 ("비활성화된 인덱스 (열)")) -> (w525:string[][])
                n265 = Replace Array Subset(array=w524, new element=w538, index (row)=53 ("비활성화된 인덱스 (열)"), index (col)=1 ("비활성화된 인덱스 (열)")) -> (w523:string[][])
                n266 = Replace Array Subset(array=w521, new element=w520, index (row)=54 ("비활성화된 인덱스 (열)"), index (col)=1 ("비활성화된 인덱스 (열)")) -> (w522:string[][])
                n267 = Replace Array Subset(array=w534, new element=w575, index (row)=48 ("비활성화된 인덱스 (열)"), index (col)=1 ("비활성화된 인덱스 (열)")) -> (w533:string[][])
                n268 = Replace Array Subset(array=w532, new element=w570, index (row)=49 ("비활성화된 인덱스 (열)"), index (col)=1 ("비활성화된 인덱스 (열)")) -> (w531:string[][])
                n269 = Replace Array Subset(array=w530, new element=w565, index (row)=50 ("비활성화된 인덱스 (열)"), index (col)=1 ("비활성화된 인덱스 (열)")) -> (w529:string[][])
                n270 = Replace Array Subset(array=w528, new element=w560, index (row)=51 ("비활성화된 인덱스 (열)"), index (col)=1 ("비활성화된 인덱스 (열)")) -> (w527:string[][])
                n271 = local write "ROM Table"(w535) -> ()
                n272 = local write "ROM Table"(w523) -> ()
                n273 = local write "ROM Table"(w522) -> ()
                n274 = local write "ROM Table"(w533) -> ()
                n275 = local write "ROM Table"(w525) -> ()
                n276 = local write "ROM Table"(w531) -> ()
                n277 = local write "ROM Table"(w529) -> ()
                n278 = local write "ROM Table"(w527) -> ()
              }
            }
          }
        }
        "Last Index" <- w9
      }
    }
    frame #2 {
      n279 = local read "ROM Table"() -> (w588:string[][])
      n280 = property class="Tbl (엄격한)"(reference=w589, "Value"=w588) -> ()  [unwired: 1 in, 2 out]
    }
  }
